vi "PYBD <-> Thingworx.vi"() -> ()   [LabVIEW 2016]
uses:
  VIs/uPythonX/uPythonX.xctl
panel:
  in  "WiFi 2":T1(xcontrol)={"VISA Refnum in"="ASRL44::INSTR", "Python Code"="import machine, network, ubinascii, ujson, urequests, utime,gc\nfrom pyb import LED\n\nWiFi = network.WLAN()\n\nmac = ubinascii.hexlify(network.WLAN().config(\"mac\"),\":\").decode()\nprint(\"MAC address: \" + mac)\ndef connect():\n     if not WiFi.isconnected():\n          print (\"Connecting ..\")\n          WiFi.active(True)\n          WiFi.connect(\"Tufts_Wireless\",\"\")\n          i=0\n          while i < 25 and not WiFi.isconnected():\n               utime.sleep_ms(200)\n               i=i+1\n          if WiFi.isconnected():\n               print (\"Connection succeeded\")\n          else:\n               print (\"Connection failed\")     \n     return WiFi.isconnected()\n\n# Thingworx\nKey = \"f3ac5fed-eef3-4e30-a17e-df46964808e8\"\n\nurlBase = \"https://ptcacademic-dev3-twx.es.thingworx.com/Thingworx/\"\n\nheaders = {\"Accept\":\"application/json\",\"Content-Type\":\"application/json\",\"AppKey\":Key}\n\ndef Put(thing, property, type, value):\n     urlValue = urlBase + 'Things/' + thing + '/Properties/*'\n     propValue = {property:value}\n     print(propValue)\n     #  assume that the tag is already created  -      urequests.put(urlTag,headers=headers,json=propName).text\n     try:\n          response = urequests.put(urlValue,headers=headers,json=propValue)\n          print(response.text)\n          response.close()\n     except Exception as e:\n          print(e)\n\ndef Get(thing, property):\n     urlValue = urlBase + 'Things/' + thing + '/Properties/' + property\n     try:\n          response = urequests.get(urlValue,headers=headers)\n          value = response.text\n          response.close()\n          # print(value)\n          data = ujson.loads(value)\n          result = data.get(\"rows\")[0].get(property)\n     except Exception as e:\n          print(e)\n          result = e\n     return result\n     \ndef Create(thing, property, type):\n     urlValue = urlBase + 'Things/' + thing + '/Services/AddPropertyDefinition'\n     propValue = {'name':property,'type':type,\"logged\":False}\n     try:\n          response = urequests.post(urlValue,headers=headers,json=propValue)\n          reply = response.text\n          response.close()\n     except:\n         reply = ''\n     return reply\n\ndef Delete(thing, property):\n     urlValue = urlBase + 'Things/' + thing + '/Services/RemovePropertyDefinition'\n     propValue = {'name':property}\n     try:\n          response = urequests.post(urlValue,headers=headers,json=propValue)\n          reply = response.text\n          response.close()\n     except:\n          reply = ''\n     return reply\n\nprint (\"WiFi: \",connect())\nPut('PTCTalk', 'Sejal', 'NUMBER',2)\nPut('PTCTalk', 'SejalText', 'STRING','a test')\nGet('PTCTalk', 'Sejal')\nGet('PTCTalk', 'SejalText')\n\nCreate('PTCTalk', 'test', 'NUMBER')\nPut('PTCTalk', 'Sejal', 'NUMBER',2)\nutime.sleep(2)\nDelete('PTCTalk', 'test')\n\n# this allows you to read and write numbers to Sejal and text to SejalText\n\n\n\n"}
  in  "WiFi":T1(xcontrol)={"VISA Refnum in"="ASRL44::INSTR", "Python Code"="import machine, network, ubinascii, ujson, urequests, utime,gc\nfrom pyb import LED\n\nWiFi = network.WLAN()\n\nmac = ubinascii.hexlify(network.WLAN().config(\"mac\"),\":\").decode()\nprint(\"MAC address: \" + mac)\ndef connect():\n     if not WiFi.isconnected():\n          print (\"Connecting ..\")\n          WiFi.active(True)\n          WiFi.connect(\"Tufts_Wireless\",\"\")\n          i=0\n          while i < 25 and not WiFi.isconnected():\n               utime.sleep_ms(200)\n               i=i+1\n          if WiFi.isconnected():\n               print (\"Connection succeeded\")\n          else:\n               print (\"Connection failed\")     \n     return WiFi.isconnected()\n\n# Thingworx\nKey = \"3b37d120-36b0-4653-ba20-b5887e055866\"\n\nurlBase = \"https://pp-1804271345f2.portal.ptc.io:8443/Thingworx/\"\n\nheaders = {\"Accept\":\"application/json\",\"Content-Type\":\"application/json\",\"AppKey\":Key}\n\ndef Put(thing, property, type, value):\n     urlValue = urlBase + 'Things/' + thing + '/Properties/*'\n     propValue = {property:value}\n     print(propValue)\n     #  assume that the tag is already created  -      urequests.put(urlTag,headers=headers,json=propName).text\n     try:\n          response = urequests.put(urlValue,headers=headers,json=propValue)\n          print(response.text)\n          response.close()\n     except Exception as e:\n          print(e)\n\ndef Get(thing, property):\n     urlValue = urlBase + 'Things/' + thing + '/Properties/' + property\n     try:\n          response = urequests.get(urlValue,headers=headers)\n          value = response.text\n          response.close()\n          # print(value)\n          data = ujson.loads(value)\n          result = data.get(\"rows\")[0].get(property)\n     except Exception as e:\n          print(e)\n          result = e\n     return result\n     \ndef Create(thing, property, type):\n     urlValue = urlBase + 'Things/' + thing + '/Services/AddPropertyDefinition'\n     propValue = {'name':property,'type':type,\"logged\":False}\n     try:\n          response = urequests.post(urlValue,headers=headers,json=propValue)\n          reply = response.text\n          response.close()\n     except:\n         reply = ''\n     return reply\n\ndef Delete(thing, property):\n     urlValue = urlBase + 'Things/' + thing + '/Services/RemovePropertyDefinition'\n     propValue = {'name':property}\n     try:\n          response = urequests.post(urlValue,headers=headers,json=propValue)\n          reply = response.text\n          response.close()\n     except:\n          reply = ''\n     return reply\n\nprint (\"WiFi: \",connect())\nPut('PTCTalk', 'Sejal', 'NUMBER',2)\nPut('PTCTalk', 'SejalText', 'STRING','a test')\nGet('PTCTalk', 'Sejal')\nGet('PTCTalk', 'SejalText')\n\nCreate('PTCTalk', 'test', 'NUMBER')\nPut('PTCTalk', 'Sejal', 'NUMBER',2)\nutime.sleep(2)\nDelete('PTCTalk', 'test')\n\n# this allows you to read and write numbers to Sejal and text to SejalText\n\n\n\n"}
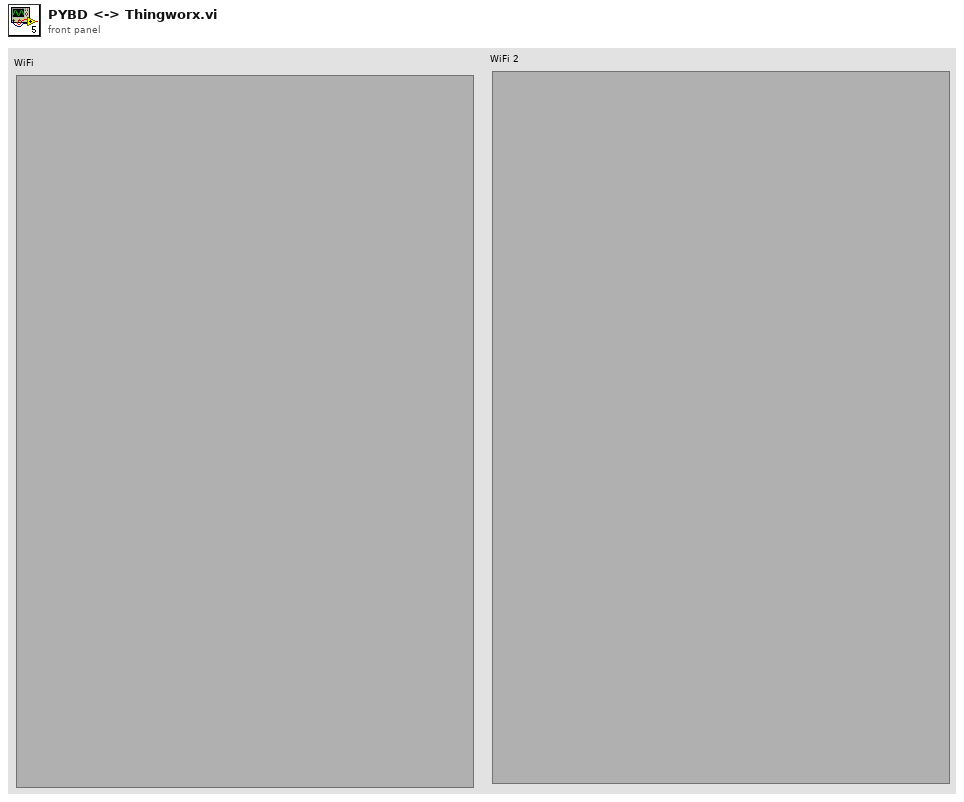
[diagram p1: front panel]
types:
  T1 = cluster{"VISA Refnum in":refnum<visa-resource-name>, "Python Code":string}
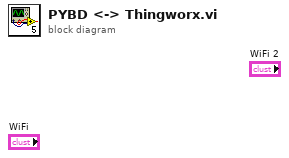
[diagram p0: block diagram]
diagram:
